vi "Real Matrix Logarithm_Real Log.vi"(11 "Input Matrix":T1) -> (0 "error":i32, 3 "Matrix Logarithm":T1)   [LabVIEW 2018, in "NI_AALBase.lvlib"]
uses:
  NI_AALBase.lvlib
  RealMatrix.ctl
  Eigenvalue Order.ctl
  Real Transpose Matrix.vi
  Real A x B.vi
  NI_AALPro.lvlib
  NI_Matrix.lvlib
  <resource>/lvanlys.dll
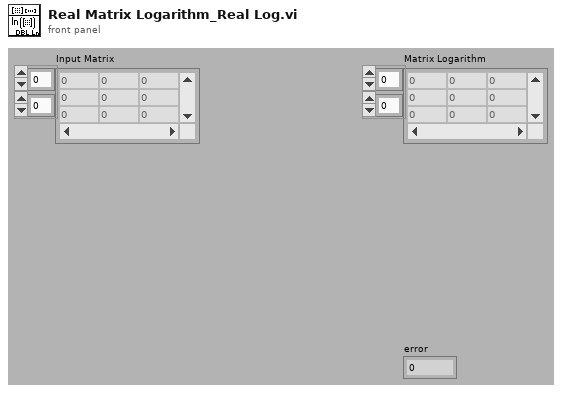
[diagram p1: front panel]
types:
  T1 = typedef "NI_Matrix.lvlib/RealMatrix.ctl" = dbl[][]
  T2 = typedef "NI_AALPro.lvlib/Eigenvalue Order.ctl" = u16
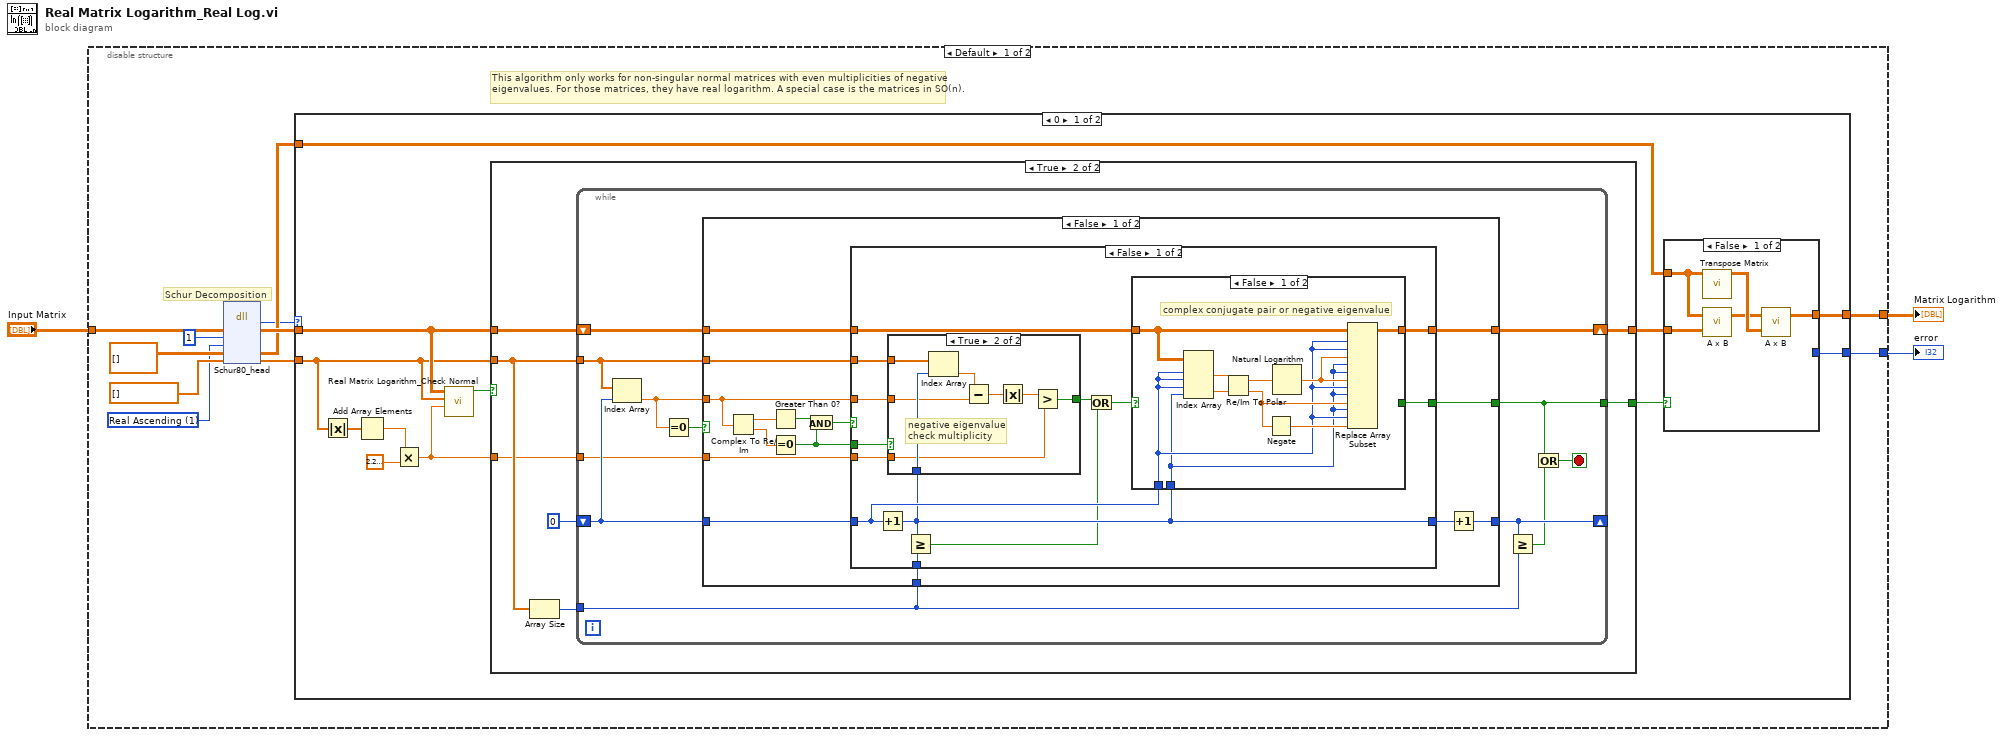
[diagram p0: block diagram]
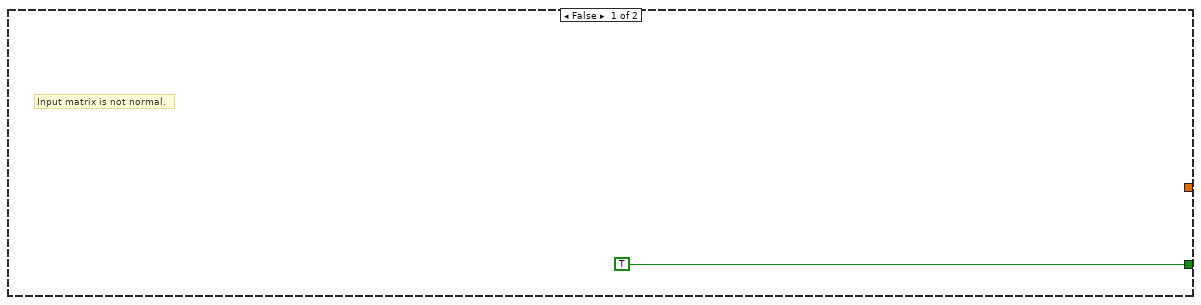
[diagram p2: hidden frame]
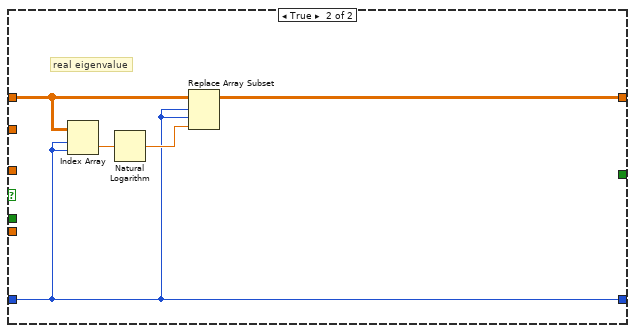
[diagram p5: hidden frame]
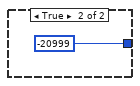
[diagram p7: hidden frame]
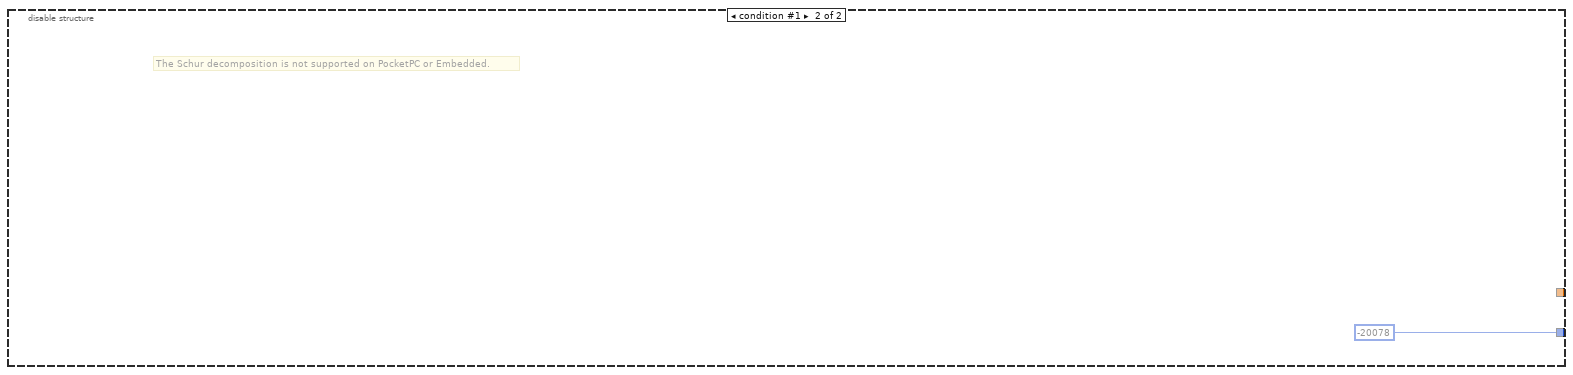
[diagram p9: hidden frame]
diagram:
  n1 = disable-structure shown="Default" {
    disable-tunnel: [w14 _] -> w3
    disable-tunnel: [w13 -20078 ("error")] -> w2
    disable-tunnel: "Input Matrix" -> [w12 _]
    frame condition #0 (active) {
      w4 = T2 1 items=["No Reorder", "Real Ascending", "Real Descending", "Magnitude Ascending", "Magnitude Descending"] ("order")
      # "Schur Decomposition"
      # "This algorithm only works for non-singular normal matrices with even multiplicities of negative eigenvalues. For those matrices, they have real logarithm. A special case is the matrices in SO(n)."
      n2 = dll-call lib="C:/Program Files (x86)/National Instruments/LabVIEW 2018/resource/lvanlys.*" fn="Schur80_head"("aH"=w12, "compSV"=1, "orderOpt"=w4, "qH"=T1 [] ("Input Matrix"), "evH"=cdb[] [] ("Eigenvalues")) -> ("return type"=w6:i32, "aH"=w11:T1, "qH"=w10:T1, "evH"=w7:cdb[])  [unwired: 5 in, 2 out]
      n3 = case shown="0" w6 {
        selector: w6 -> [_ w109]
        tunnel: w11 -> [w20 _]
        tunnel: w10 -> [w24 _]
        tunnel: w7 -> [w19 _]
        tunnel: [w23 _] -> w14
        tunnel: [w22 w109] -> w13
        frame 0 {
          n4 = Absolute Value(x=w19) -> (abs(x)=w18:dbl[])
          n5 = Add Array Elements(numeric array=w18) -> (sum=w17:dbl)
          n6 = Multiply(x=w17, y=2.220446049250313e-16) -> (x*y=w15:dbl)
          n7 = call "Real Matrix Logarithm_Check Normal.vi"("tolerance"=w15, "Eigenvalues"=w19, "Schur Form"=w20) -> ("normal?"=w21:bool)  [unwired: 8 in]
          n8 = case shown="True" w21 {
            tunnel: w20 -> [_ w34]
            tunnel: w19 -> [_ w32]
            tunnel: [TRUE w30] -> w26
            tunnel: [_ w29] -> w25
            tunnel: w15 -> [_ w28]
            frame False {
              # "Input matrix is not normal."
            }
            frame True {
              n9 = Array Size(array=w32) -> (size(s)=w31:i32)
              n10 = while {
                tunnel: w32 -> [w41]
                shift-right: [w40] -> _
                shift-left: 0 -> [w45]
                shift-right: [w44] -> w29
                shift-left: w34 -> [w46]
                tunnel: w31 -> [w39]
                tunnel: [w36] -> w30
                tunnel: w28 -> [w35]
                stop <- w37 stop-if-true
                n11 = Index Array(array=w41, index=w45) -> (element=w43:cdb)
                n12 = Equal To 0?(x=w43) -> (x = 0?=w42:bool)
                n13 = case shown="False" w42 {
                  selector: w42 -> [_ w100]
                  tunnel: w46 -> [w60 w102]
                  tunnel: w45 -> [w59 w101]
                  tunnel: [w58 w102] -> w44
                  tunnel: w43 -> [w51 _]
                  tunnel: [w53 w101] -> w40
                  tunnel: w41 -> [w52 _]
                  tunnel: [w49 w100] -> w36
                  tunnel: w39 -> [w48 _]
                  tunnel: w35 -> [w47 _]
                  frame False {
                    n14 = Complex To Re/Im(x + iy=w51) -> (x=w57:dbl, y=w61:dbl)
                    n15 = Greater Than 0?(x=w57) -> (x > 0?=w56:bool)
                    n16 = Equal To 0?(x=w61) -> (x = 0?=w50:bool)
                    n17 = And(x=w56, y=w50) -> (x .and. y?=w55:bool)
                    n18 = case shown="False" w55 {
                      tunnel: w60 -> [w74 w98]
                      tunnel: w59 -> [w71 w95]
                      tunnel: [w73 w97] -> w58
                      tunnel: [w67 w95] -> w54
                      tunnel: w52 -> [w72 _]
                      tunnel: w51 -> [w69 _]
                      tunnel: w50 -> [w70 _]
                      tunnel: [w68 _] -> w49
                      tunnel: w48 -> [w66 _]
                      tunnel: w47 -> [w62 _]
                      frame False {
                        n19 = Increment(x=w71) -> (x+1=w67:i32)
                        n20 = case shown="True" w70 {
                          tunnel: w72 -> [_ w94]
                          tunnel: w67 -> [_ w93]
                          tunnel: w69 -> [_ w91]
                          tunnel: [_ w88] -> w65
                          tunnel: w62 -> [_ w87]
                          frame False {
                          }
                          frame True {
                            # "negative eigenvalue\ncheck multiplicity"
                            n21 = Index Array(array=w94, index=w93) -> (element=w92:cdb)
                            n22 = Subtract(x=w92, y=w91) -> (x-y=w90:cdb)
                            n23 = Absolute Value(x=w90) -> (abs(x)=w89:dbl)
                            n24 = Greater?(x=w89, y=w87) -> (0:w88:bool)
                          }
                        }
                        n25 = Greater Or Equal?(x=w67, y=w66) -> (x >= y?=w64:bool)
                        n26 = Or(x=w65, y=w64) -> (x .or. y?=w63:bool)
                        n27 = case shown="False" w63 {
                          selector: w63 -> [_ w85]
                          tunnel: w74 -> [w81 w86]
                          tunnel: [w80 w86] -> w73
                          tunnel: w71 -> [w76 _]
                          tunnel: w67 -> [w75 _]
                          tunnel: [_ w85] -> w68
                          frame False {
                            # "complex conjugate pair or negative eigenvalue"
                            n28 = Index Array(array=w81, index (row) #1=w76, index (col) #1=w76, index (row) #2=w76, index (col) #2=w75) -> (element #1=w83:dbl, element #2=w82:dbl)
                            n29 = Re/Im To Polar(2:w82, 3:w83) -> (0:w78:dbl, 1:w84:dbl)
                            n30 = Negate(x=w78) -> (-x=w77:dbl)
                            n31 = Natural Logarithm(1:w84) -> (0:w79:dbl)
                            n32 = Replace Array Subset(array=w81, new element #1=w79, index (row) #1=w76, index (col) #1=w76, new element #2=w79, index (row) #2=w75, index (col) #2=w75, new element #3=w78, index (row) #3=w76, index (col) #3=w75, new element #4=w77, index (row) #4=w75, index (col) #4=w76) -> (w80:T1)
                          }
                          frame True {
                          }
                        }
                      }
                      frame True {
                        # "real eigenvalue"
                        n33 = Index Array(array=w98, index (row)=w95, index (col)=w95) -> (element=w99:dbl)
                        n34 = Natural Logarithm(1:w99) -> (0:w96:dbl)
                        n35 = Replace Array Subset(array=w98, new element=w96, index (row)=w95, index (col)=w95) -> (w97:T1)
                      }
                    }
                    n36 = Increment(x=w54) -> (x+1=w53:i32)
                  }
                  frame True {
                    # "singular input"
                  }
                }
                n37 = Greater Or Equal?(x=w40, y=w39) -> (x >= y?=w38:bool)
                n38 = Or(x=w36, y=w38) -> (x .or. y?=w37:bool)
              }
            }
          }
          n39 = case shown="False" w26 {
            tunnel: w25 -> [w107 _]
            tunnel: w24 -> [w105 _]
            tunnel: [w106 _] -> w23
            tunnel: [_ -20999] -> w22
            frame False {
              n40 = call-poly "Transpose Matrix.vi"("Input Matrix"=w105) -> ("Matrix Transpose"=w104:T1)  [unwired: 9 in, 1 out]
              n41 = call-poly "A x B.vi"("B"=w107, "A"=w105) -> ("A x B"=w103:T1)  [unwired: 1 out]
              n42 = call-poly "A x B.vi"("B"=w104, "A"=w103) -> ("A x B"=w106:T1)  [unwired: 1 out]
            }
            frame True {
            }
          }
        }
        frame -1, Default {
        }
      }
    }
    frame condition #1 {
      # "The Schur decomposition is not supported on PocketPC or Embedded."
    }
  }
  "Matrix Logarithm" <- w3
  "error" <- w2
